vi "Kamarga_ME473_Project3_calibrationAndRolldown.vi"() -> ()   [LabVIEW 2018]
doc: "This VI demonstrates how a signal can be extracted from bandlimited noise using the filter VIs."
uses:
  <vilib>/express/express signal manip/GetorSetDDTAttributes/Shared VIs/TimeType.ctl
  <vilib>/express/express signal manip/GetorSetDDTAttributes/Shared VIs/TimeMode Enum to Boolean.vi
  <vilib>/express/express shared/transition.llb/Dynamic To Waveform Array.vi
  <vilib>/express/express signal manip/GetorSetDDTAttributes/Set DDT Attributes/SetT0.vi
  <vilib>/express/express shared/transition.llb/Waveform Array To Dynamic.vi
  <vilib>/Analysis/3filter.llb/Butterworth Filter (DBL).vi
  <vilib>/Waveform/WDTOps.llb/WDT Get Waveform Time Array DBL.vi
  <vilib>/express/express signal manip/GetorSetDDTAttributes/Set DDT Attributes/Set DDT Properties.xnode
  <vilib>/express/express signal manip/GetorSetDDTAttributes/Shared VIs/GetSetShared.lvlib
  <vilib>/Analysis/NI_AALBase.lvlib
panel:
  out "XY Graph":cluster{dbl[], "Y":dbl[]}[](graph)
  in  "MyDAQ Device Name":tag="myDAQ3"
  in  "Duration (sec)":i32=5
  in  "Samples per sec":dbl=1000.0
  out "Waveform Graph":dynamicdata(graph) caption="data"
  # "ME 473\nBall-on-Track Experiment\nBall-on-Track #4"
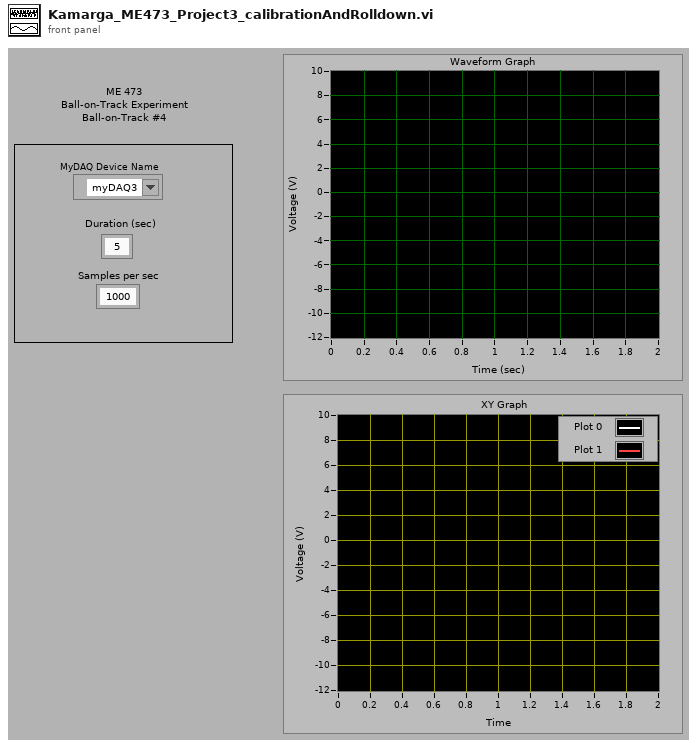
[diagram p1: front panel]
types:
  T1 = typedef "GetSetShared.lvlib/TimeType.ctl" = enum16{"Absolute", "Relative"}
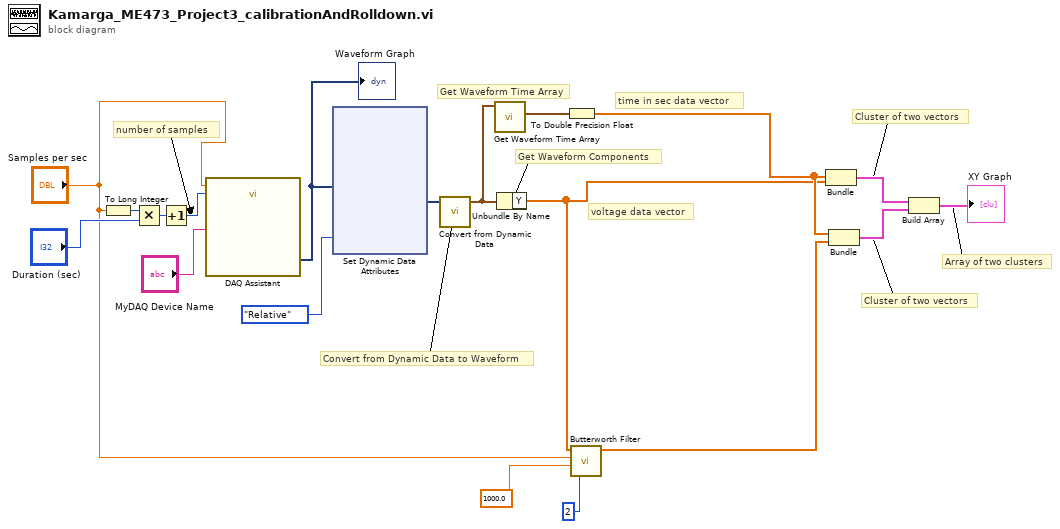
[diagram p0: block diagram]
diagram:
  # "Array of two clusters"
  # "Cluster of two vectors"
  # "Cluster of two vectors"
  # "Get Waveform Components"
  # "Convert from Dynamic Data to Waveform"
  # "Get Waveform Time Array"
  # "time in sec data vector"
  # "voltage data vector"
  # "number of samples"
  n1 = To Long Integer(number="Samples per sec") -> (32bit integer=w19:i32)
  n2 = Multiply(x=w19, y="Duration (sec)") -> (x*y=w17:i32)
  n3 = Increment(x=w17) -> (x+1=w16:i32)
  n4 = call "DAQ Assistant"("rate"="Samples per sec", "number of samples"=w16, "device name"="MyDAQ Device Name") -> ("data"=w14:dynamicdata)  [unwired: 14 in, 2 out]
  "Waveform Graph" <- w14
  n5 = xnode "Set Dynamic Data Attributes"("Signals In"=w14, "Time Mode"=TimeType."Relative") -> ("Signals Out"=w13:dynamicdata)  [unwired: 2 in, 1 out]
  n6 = call "Convert from Dynamic Data"("Dynamic Data Type"=w13) -> ("Waveform"=w10:waveform(dbl))  [unwired: 3 in]
  n7 = call-poly <vilib>:"Get Waveform Time Array.vi"("waveform in"=w10) -> ("X array"=w12:timestamp[])  [unwired: 9 in, 1 out]
  n8 = Unbundle By Name ("Get Waveform Components")(w10) -> ("Y"=w4:dbl[])
  n9 = To Double Precision Float(number=w12) -> (double precision float=w9:dbl[])
  n10 = call-poly <vilib>:"Butterworth Filter.vi"("order"=2, "high cutoff freq: fh"=1000.0, "sampling freq: fs"="Samples per sec", "X"=w4) -> ("Filtered X"=w3:dbl[])  [unwired: 4 in, 1 out]
  n11 = Bundle "Bundle"(w9, "Y"=w4) -> (w8:cluster{dbl[], "Y":dbl[]})  [unwired: 1 in]
  n12 = Bundle "Bundle"(w9, "Filtered X"=w3) -> (w7:cluster{dbl[], "Filtered X":dbl[]})  [unwired: 1 in]
  n13 = Build Array "Build Array"(w8, w7) -> (→"XY Graph":cluster{dbl[], "Filtered X":dbl[]}[])
